vi "ModifyStandby.vi"(0 "Center":cluster{dbl, dbl, dbl}, 1 "StandbyArray In":dbl[](array[numeric])) -> (2 "StandbyArray Out":dbl[](array[numeric]))   [LabVIEW 2014]
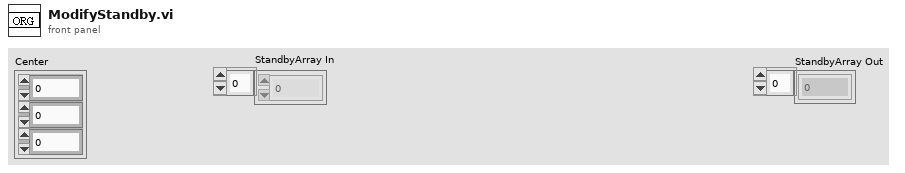
[diagram p1: front panel]
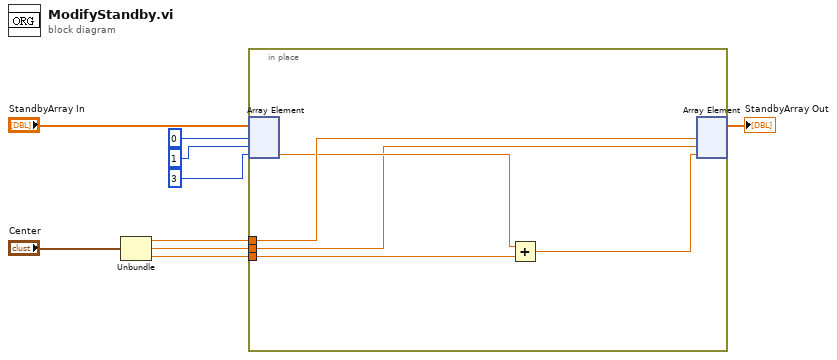
[diagram p0: block diagram]
diagram:
  n1 = Unbundle("Center") -> (w4:dbl, w2:dbl, w3:dbl)
  n2 = in-place {
    in-place-border: w4 -> [w14]
    in-place-border: w3 -> [w11]
    in-place-border: w2 -> [w10]
    n3 = in-place-array #1("StandbyArray In", 0, 1, 3) -> (w13:dbl)  [unwired: 2 out]
    n4 = Add(x=w13, y=w11) -> (x+y=w12:dbl)
    n5 = in-place-array #1(w14, w10, w12) -> (→"StandbyArray Out":dbl[])  [unwired: 3 out]
  }
